vi "8bitTo16bit.vi"(0 "input_byte":u8[](array[numeric])) -> (1 "output_int16":i32[](array[numeric]), 2 "cell":u8[](array[numeric]))   [LabVIEW 2013]
panel:
  # "The input of this VI is a byte vector of 8 indexes, that contains 4 uint16_t separeted into 2 bytes in the vector.\nEach two bytes represent a number os 16 bits, where the fist bite is the LSB and the second ins MSB"
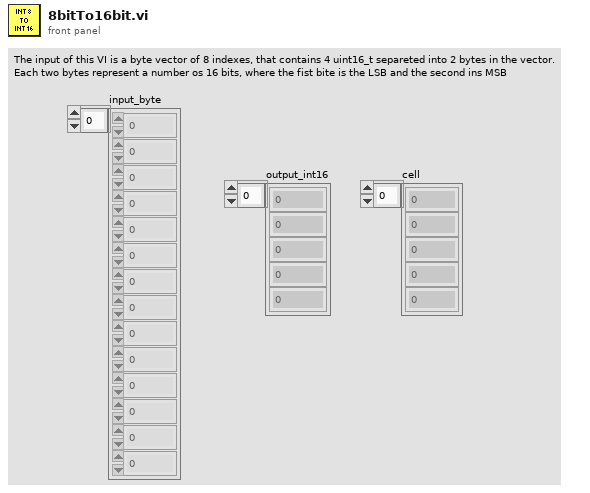
[diagram p1: front panel]
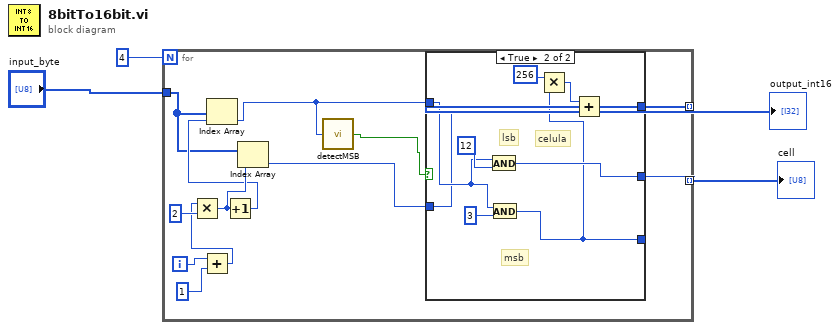
[diagram p0: block diagram]
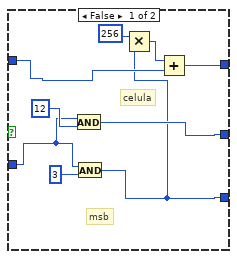
[diagram p2: hidden frame]
diagram:
  n1 = for {
    N: 4 -> [_]
    tunnel: "input_byte" -> [w12]
    tunnel: [w15] -> w3 mode=indexing
    tunnel: [w10] -> w1 mode=indexing
    i -> [w6]
    n2 = Add(x=w6, y=1) -> (x+y=w5:i32)
    n3 = Multiply(x=w5, y=2) -> (x*y=w14:i32)
    n4 = Increment(x=w14) -> (x+1=w13:i32)
    n5 = Index Array(array=w12, index=w13) -> (element=w9:u8)
    n6 = Index Array(array=w12, index=w14) -> (element=w11:u8)
    n7 = call "detectMSB.vi"("dataInput"=w9) -> ("result"=w8:bool)
    n8 = case shown="True" w8 {
      tunnel: [w21 w32] -> w15
      tunnel: w11 -> [w18 w27]
      tunnel: [w20 w29] -> w10
      tunnel: [w17 w26] -> _
      tunnel: w9 -> [w19 w28]
      frame False {
        # "celula"
        # "msb"
        n9 = And(x=w18, y=u8 12) -> (x .and. y?=w20:u8)
        n10 = And(x=w18, y=u8 3) -> (x .and. y?=w17:u8)
        n11 = Multiply(x=256, y=w17) -> (x*y=w24:i32)
        n12 = Add(x=w24, y=w19) -> (x+y=w21:i32)
      }
      frame True {
        # "lsb"
        # "celula"
        # "msb"
        n13 = And(x=w28, y=u8 12) -> (x .and. y?=w29:u8)
        n14 = And(x=w28, y=u8 3) -> (x .and. y?=w26:u8)
        n15 = Multiply(x=256, y=w26) -> (x*y=w33:i32)
        n16 = Add(x=w33, y=w27) -> (x+y=w32:i32)
      }
    }
  }
  "output_int16" <- w3
  "cell" <- w1
